vi "Kinematics_Pose2d_TransformBy.vi"(9 "Other TRANSFORM":T4 {"ROTATION"."SIN" format="%13.4f"; "ROTATION"."COS" format="%13.4f"; "ROTATION"."VALUE" format="%13.4f"; "TRANSLATION"."Y" format="%14.3f"; "TRANSLATION"."X" format="%14.3f"}, 11 "In POSE":T1 {"ROTATION"."SIN" format="%13.4f"; "ROTATION"."COS" format="%13.4f"; "ROTATION"."VALUE" format="%13.4f"; "TRANSLATION"."Y" format="%14.3f"; "TRANSLATION"."X" format="%14.3f"}) -> (3 "Out POSE Out":T1 {"ROTATION"."SIN" format="%13.4f"; "ROTATION"."COS" format="%13.4f"; "ROTATION"."VALUE" format="%13.4f"; "TRANSLATION"."Y" format="%14.3f"; "TRANSLATION"."X" format="%14.3f"})   [LabVIEW 2020, in "Swerve_Odometry_SEN.lvlib"]
doc: "Transforms the pose by the given transformation and returns the new transformed pose. \"plus\" is the same as \"transformBy\"\n\nThe matrix multiplication is as follows\n [x_new] [cos, -sin, 0][transform.x]\n [y_new] += [sin, cos, 0][transform.y]\n [t_new] [0, 0, 1][transform.t]\n\nParameters:\n - IN POSE - The input POSE data structure\n - OTHER TRANSFORM - The transform to transform the pose by.\n\nReturn:\n - OUT POSE - The transformed pose."
uses:
  Swerve_Odometry_SEN.lvlib
  Cluster_TRANSLATION2D.ctl
  Cluster_POSE2D.ctl
  Cluster_ROTATION2D.ctl
  Cluster_TRANSFORM2D.ctl
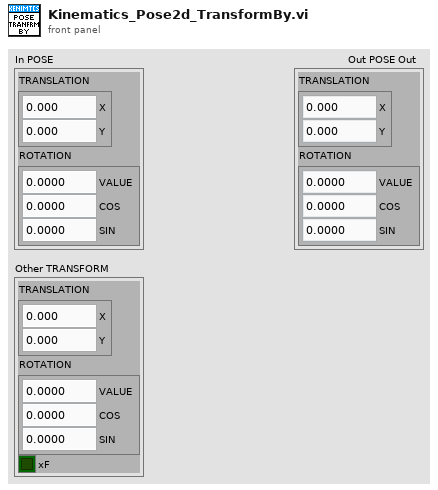
[diagram p1: front panel]
types:
  T1 = typedef "Swerve_Odometry_SEN.lvlib/Cluster_POSE2D.ctl" = cluster{"TRANSLATION":T2, "ROTATION":T3}
  T2 = typedef "Swerve_Odometry_SEN.lvlib/Cluster_TRANSLATION2D.ctl" = cluster{"X":dbl, "Y":dbl}
  T3 = typedef "Swerve_Odometry_SEN.lvlib/Cluster_ROTATION2D.ctl" = cluster{"VALUE":dbl, "COS":dbl, "SIN":dbl}
  T4 = typedef "Swerve_Odometry_SEN.lvlib/Cluster_TRANSFORM2D.ctl" = cluster{"TRANSLATION":T2, "ROTATION":T3, "xF":bool}
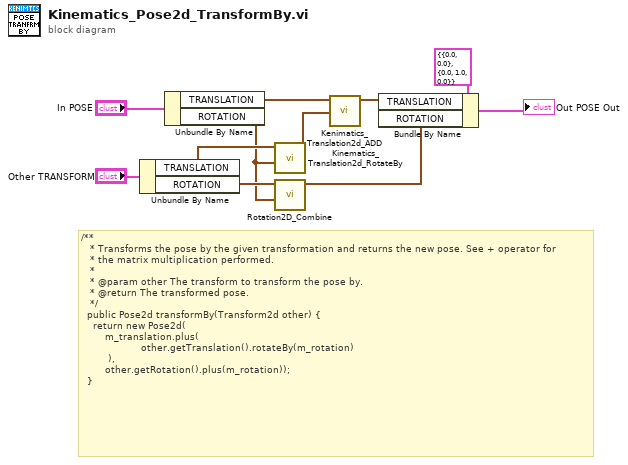
[diagram p0: block diagram]
diagram:
  # "/**\n   * Transforms the pose by the given transformation and returns the new pose. See + operator for\n   * the matrix multiplication performed.\n   *\n   * @param other The transform to transform the pose by.\n   * @return The transformed pose.\n   */\n  public Pose2d transformBy(Transform2d other) {\n    return new Pose2d(\n        m_translation.plus(\n\t\t                  other.getTranslation().rotateBy(m_rotation)\n\t        ),\n        other.getRotation().plus(m_rotation));\n  }"
  n1 = Unbundle By Name("Other TRANSFORM") -> ("TRANSLATION"=w9:T2, "ROTATION"=w6:T3)
  n2 = Unbundle By Name("In POSE") -> ("TRANSLATION"=w7:T2, "ROTATION"=w5:T3)
  n3 = call "Kinematics_Translation2d_RotateBy.vi"("other Rotation"=w5, "In Translation"=w9) -> ("Out Translation"=w8:T2)  [unwired: 9 in]
  n4 = call "Rotation2D_Combine.vi"("other Rotation"=w5, "in ROTATION"=w6) -> ("out ROTATION"=w2:T3)  [unwired: 9 in]
  n5 = call "Kenimatics_Translation2d_ADD.vi"("Other Translation"=w8, "In Translation"=w7) -> ("Out Translation Out"=w3:T2)  [unwired: 9 in]
  n6 = Bundle By Name(cluster=T1 {"TRANSLATION"={"X"=0.0, "Y"=0.0}, "ROTATION"={"VALUE"=0.0, "COS"=1.0, "SIN"=0.0}} ("POSE"), "TRANSLATION"=w3, "ROTATION"=w2) -> (→"Out POSE Out":T1)
